vi "Main.vi"() -> ()   [LabVIEW 2020]
uses:
  <vilib>/Utility/error.llb/DialogType.ctl
  Controls/Core def.ctl
  Controls/JSON image def.ctl
  Controls/State Def.ctl
  Controls/Icons def.ctl
  <vilib>/vision/Image Controls.llb/IMAQ Image.ctl
  <vilib>/vision/NI_Vision_Development_Module.lvlib
panel:
  out "Image":T1(plugin-control)
  in  "Baud":u32=115200
  in  "Port":refnum<visa-resource-name>="COM6"
  out "STM Feedback":string
  in  "Stop filter":bool
  in  "Stop process":bool
  in  "Filter":bool
  in  "Process":bool
  in  "Stop acquisition":bool
  in  "Acquire":bool
  in  "Stop program":bool
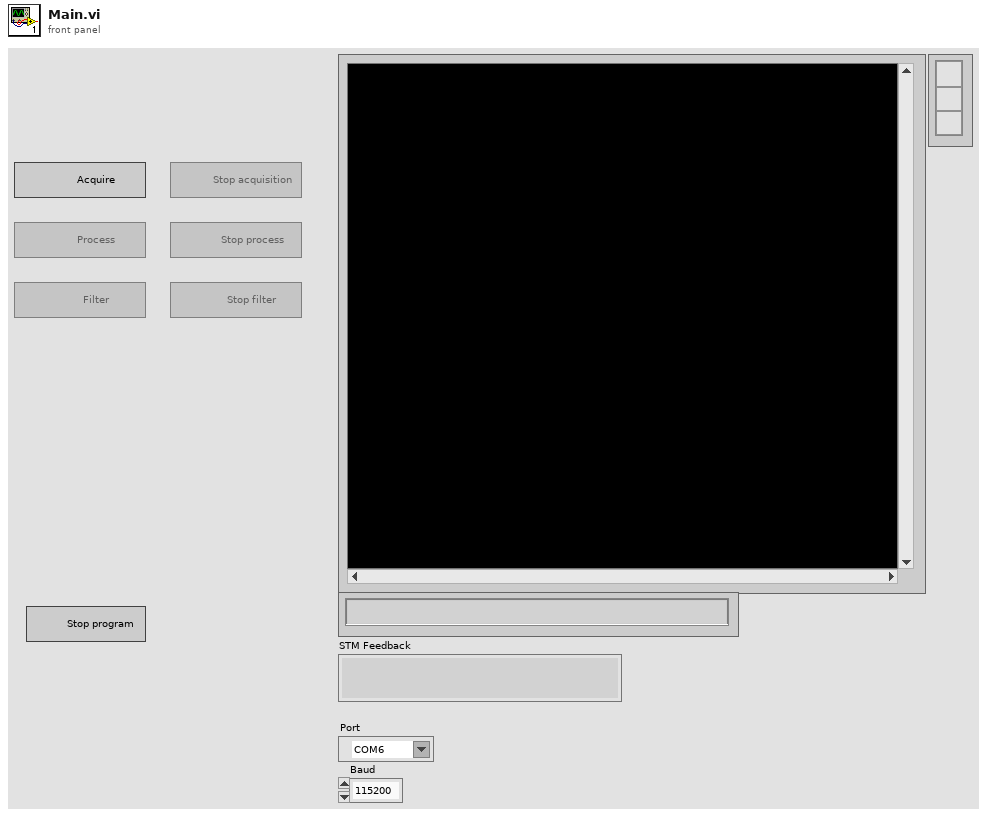
[diagram p1: front panel]
types:
  T1 = typedef "IMAQ Image.ctl" = refnum<image>
  T2 = typedef "DialogType.ctl" = u16
  T3 = enum32{"Invalid", "Standard", "Closed", "Hidden", "Minimized", "Maximized"}
  T4 = enum32{"invalid app kind", "Development System", "Run Time System", "Student Edition", "Embedded LabVIEW", "Evaluation", "Custom"}
  T5 = typedef "Icons def.ctl" = cluster{"Acquire":refnum<vi>, "Process":refnum<vi>, "Filter":refnum<vi>, "Stop acquisition":refnum<vi>, "Stop process":refnum<vi>, "Stop filter":refnum<vi>}
  T6 = typedef "State Def.ctl" = cluster{"Acquisition":bool, "Processing":bool, "Filtering":bool}
  T7 = typedef "JSON image def.ctl" = cluster{"Image Pixels (U8)":u8[][], "Image Pixels (U8) 2":u8[][], "Image Pixels (U8) 3":u8[][], "element":i32}
  T8 = typedef "Core def.ctl" = cluster{"Current VI Reference":refnum<vi>, "Close Panel on Exit?":bool}
  T9 = cluster{"Core":T8, "State":T6, "Icons":T5, "Color":i32, "New Image":T1, "JSON string":string}
  T10 = typedef "Image Type" = u32
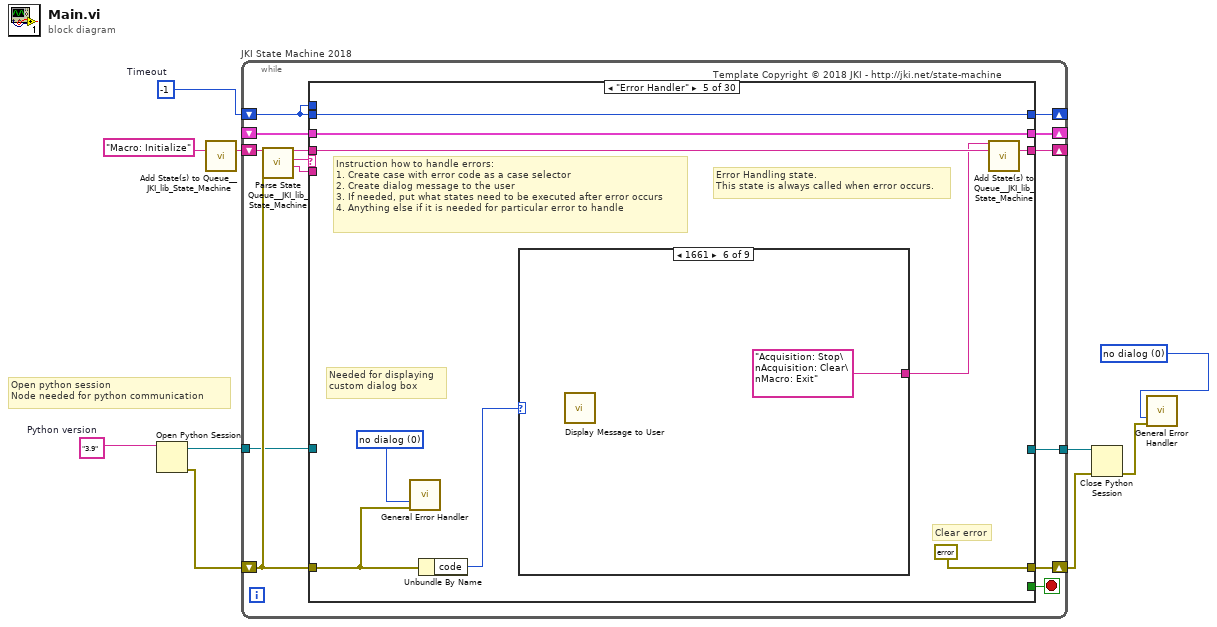
[diagram p0: block diagram]
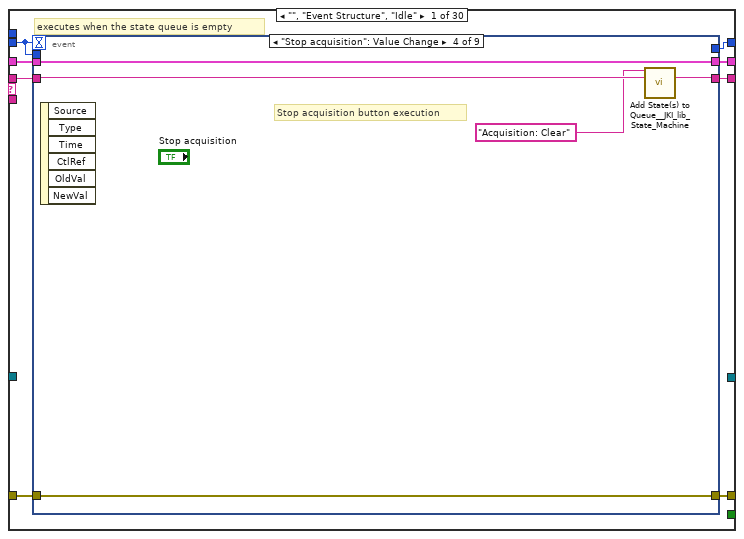
[diagram p2: hidden frame]
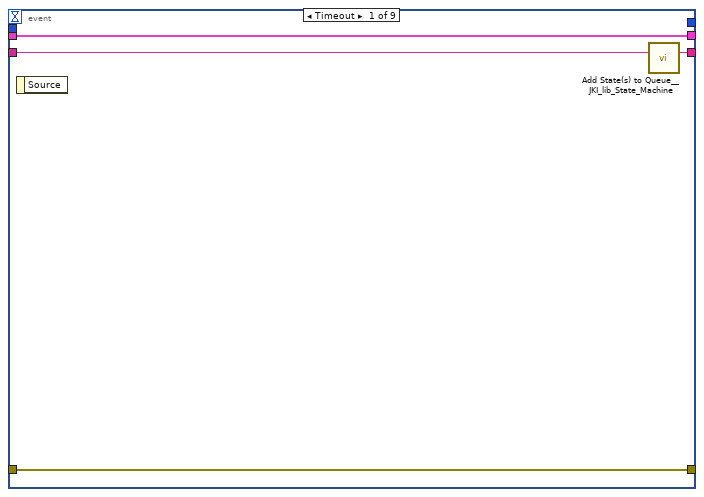
[diagram p3: hidden frame]
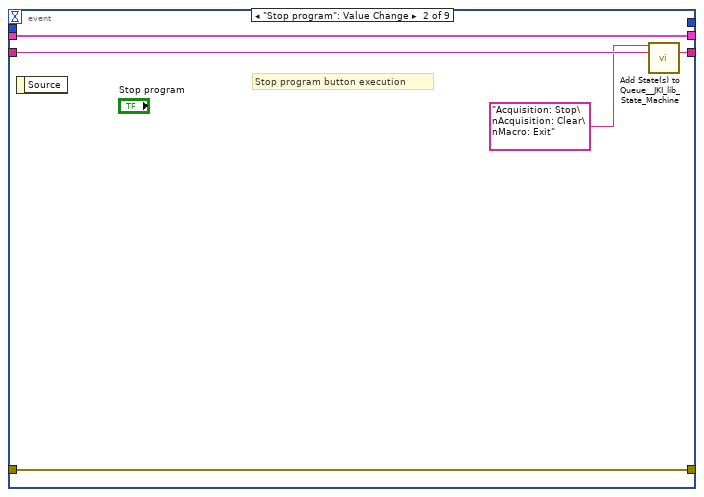
[diagram p4: hidden frame]
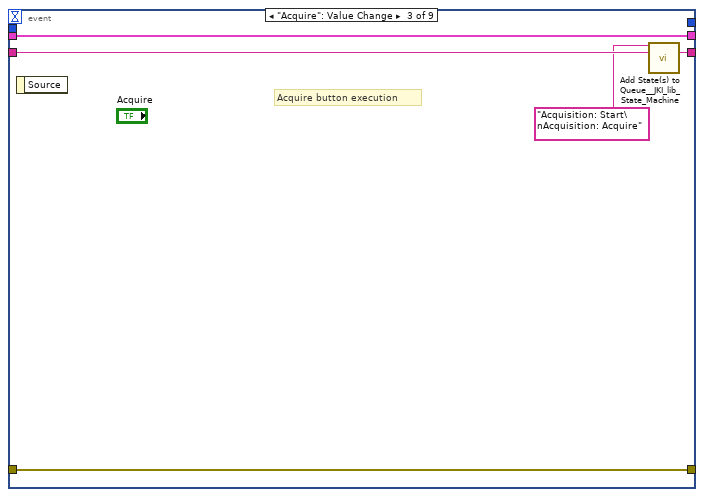
[diagram p5: hidden frame]
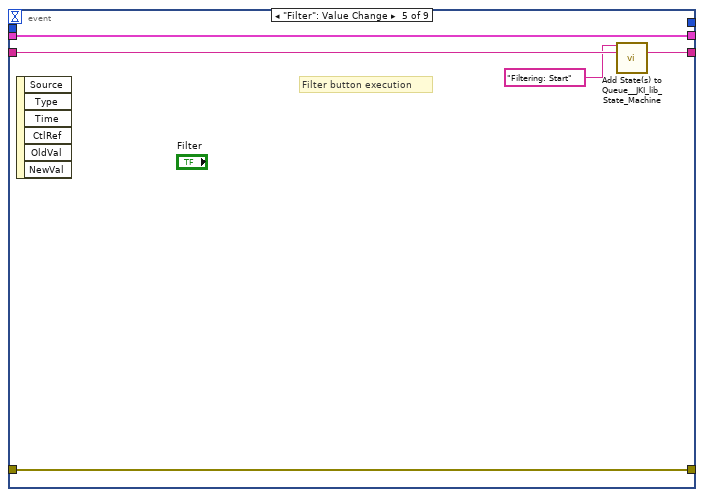
[diagram p6: hidden frame]
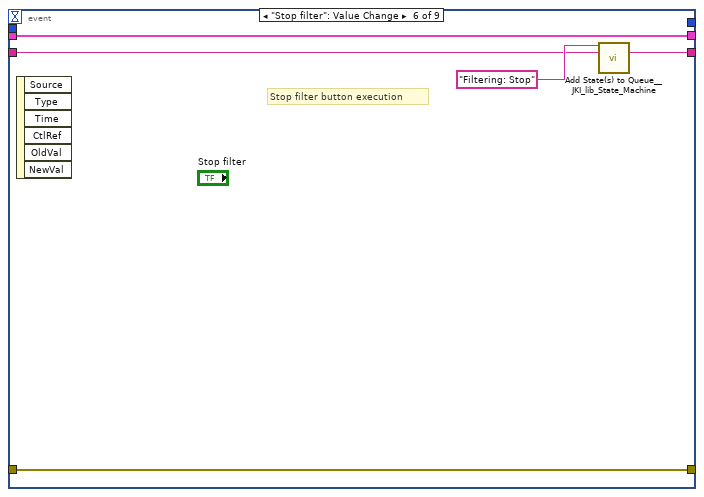
[diagram p7: hidden frame]
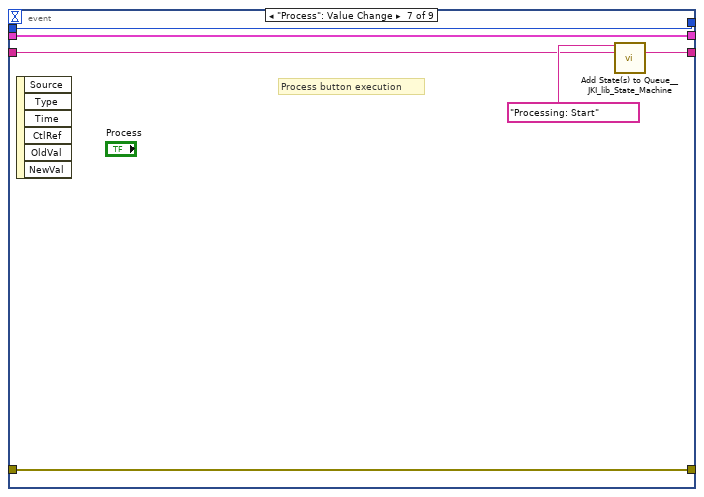
[diagram p8: hidden frame]
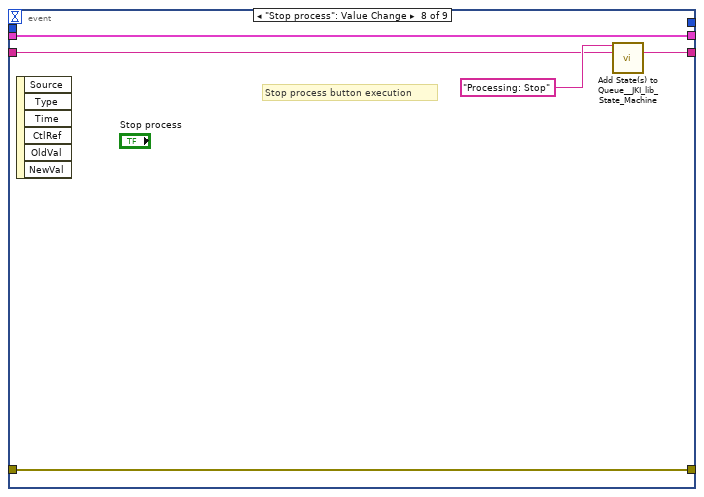
[diagram p9: hidden frame]
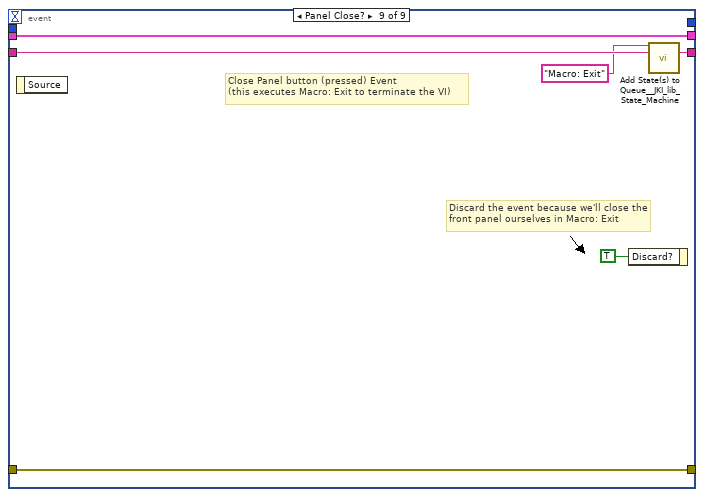
[diagram p10: hidden frame]
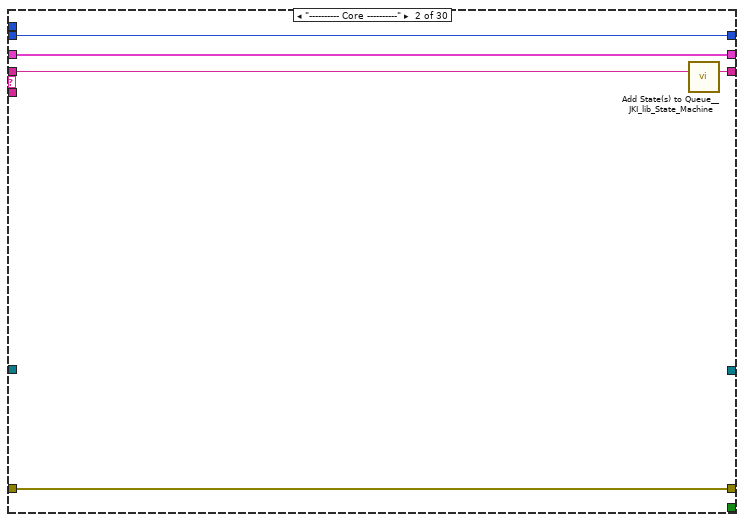
[diagram p11: hidden frame]
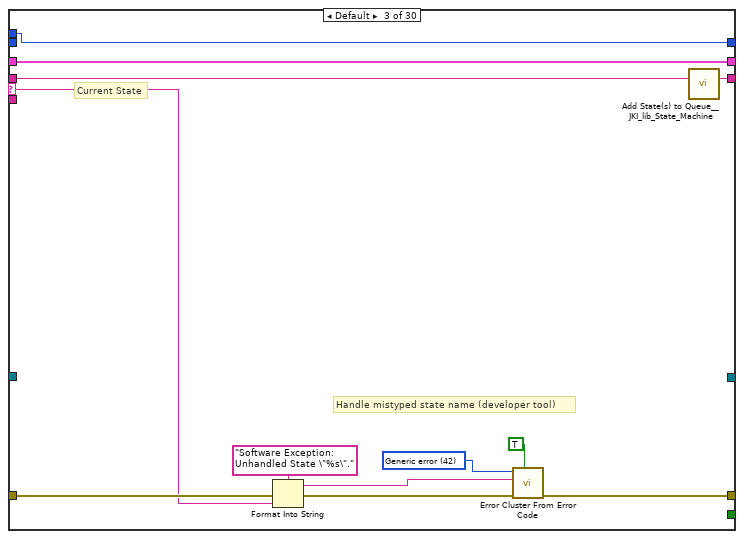
[diagram p12: hidden frame]
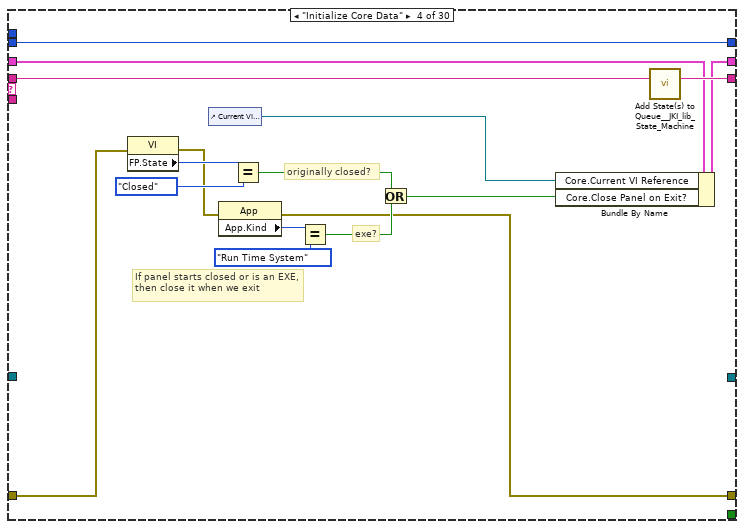
[diagram p13: hidden frame]
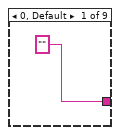
[diagram p14: hidden frame]
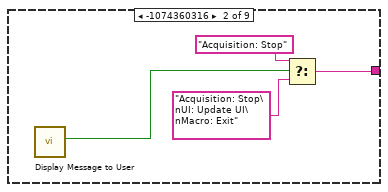
[diagram p15: hidden frame]
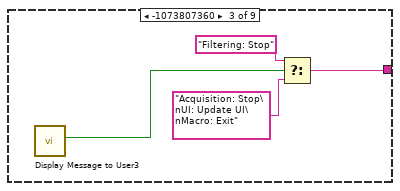
[diagram p16: hidden frame]
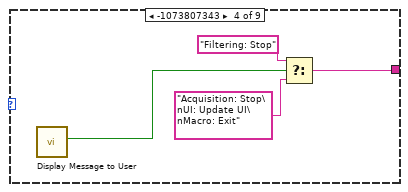
[diagram p17: hidden frame]
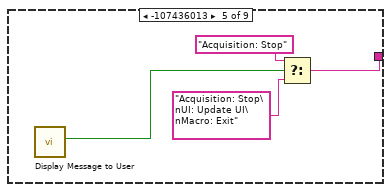
[diagram p18: hidden frame]
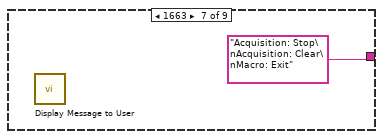
[diagram p19: hidden frame]
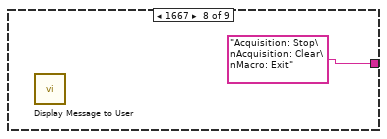
[diagram p20: hidden frame]
diagram:
  w2 = T2 0 items=["no dialog", "OK message", "continue or stop message", "OK message + warnings", "continue/stop + warnings"] ("type of dialog (OK msg:1)")
  w6 = "3.9"  # Python version
  w8 = -1  # Timeout
  # "Open python session\nNode needed for python communication"
  n1 = Open Python Session(python version=w6) -> (session out=w7:refnum<k35>, error out=w5:errorcluster)  [unwired: 2 in]
  n2 = call <vilib>:"Add State(s) to Queue__JKI_lib_State_Machine.vi"("State(s) in (\"\")"="Macro: Initialize") -> ("States Out"=w10:string)  [unwired: 14 in]
  n3 = while "JKI State Machine 2018" {
    shift-right: [w17] -> _
    shift-left: _ -> [w16]
    shift-right: [w20] -> w4
    shift-left: w5 -> [w15]
    shift-right: [w19] -> _
    shift-left: w10 -> [w21]
    shift-right: [w14] -> _
    shift-left: w8 -> [w13]
    tunnel: w7 -> [w12]
    tunnel: [w11] -> w3
    stop <- w18 stop-if-true
    # "Template Copyright © 2018 JKI - http://jki.net/state-machine"
    n4 = call <vilib>:"Parse State Queue__JKI_lib_State_Machine.vi"("State Queue"=w21, "Error In (no error)"=w15) -> ("Remaining States"=w23:string, "Current State"=w24:string, "Arguments"=w22:string)  [unwired: 11 in]
    n5 = case shown="\"Error Handler\"" w24 {
      selector: w24 -> [_ _ w85 _ _ _ _ _ _ _ _ _ _ _ _ _ _ _ _ _ _ _ _ _ _ _ _ _ _ _]
      tunnel: w23 -> [w32 w83 w89 w111 w120 w151 w156 w178 w185 w190 w205 w214 w221 w233 w298 w304 w315 w320 w334 w353 w372 w381 w386 w400 w413 w429 w434 w447 w458 w471]
      tunnel: w22 -> [_ _ _ _ _ _ _ _ _ _ _ _ w216 w227 _ _ _ _ _ _ _ _ _ _ _ _ _ _ _ _]
      tunnel: w16 -> [w30 w80 w87 w105 w117 w149 w153 _ w181 w187 w201 w207 w219 w229 w295 w301 w312 w317 w330 w351 w368 w377 w383 w397 w410 w425 w431 w443 w455 w466]
      tunnel: [w29 w81 w91 w96 errorcluster {"status"=FALSE, "code"=0, "source"=""} ("error out") w148 w154 w167 w182 w188 w203 w212 w217 w230 w296 w302 w313 w318 w332 w339 w370 w379 w384 w387 w406 w427 w432 w445 w448 w469] -> w20
      tunnel: w15 -> [w28 w81 w90 w98 w114 w148 w154 w172 w183 w188 w203 w212 w218 w231 w296 w302 w313 w318 w332 w349 w370 w379 w384 w387 w407 w427 w432 w445 w449 w469]
      tunnel: [w31 w82 w88 w110 w119 w150 w155 w177 w184 w189 w204 w213 w220 w232 w297 w303 w314 w319 w333 w352 w371 w380 w385 w399 w412 w428 w433 w446 w457 w470] -> w19
      tunnel: [_ _ _ _ _ TRUE _ _ _ _ _ _ _ _ _ _ _ _ _ _ _ _ _ _ _ _ _ _ _ _] -> w18
      tunnel: [w27 w80 w87 w109 w117 w149 w153 w157 w181 w187 w201 w207 w219 w229 w295 w301 w312 w317 w328 w343 w354 w377 w383 w395 w409 w422 w431 w435 w455 w459] -> w17
      tunnel: w13 -> [w25 w79 _ w100 w116 w146 w152 w174 w180 w186 w202 w211 w215 w226 w294 w299 w306 w316 w329 w350 w369 w378 w382 w398 w411 w426 w430 w444 w456 w468]
      tunnel: [w26 w79 w84 w100 w116 w146 w152 w174 w180 w186 w202 w211 w215 w226 w294 w299 w306 w316 w329 w350 w369 w378 w382 w398 w411 w426 w430 w444 w456 w468] -> w14
      tunnel: w13 -> [_ _ w84 _ _ _ _ _ _ _ _ _ _ _ _ _ _ _ _ _ _ _ _ _ _ _ _ _ _ _]
      tunnel: w12 -> [_ _ _ _ _ w145 _ _ _ _ _ _ _ _ _ _ _ _ _ _ _ _ _ _ w408 _ _ _ _ _]
      tunnel: [_ _ _ _ _ w145 _ _ _ _ _ _ _ _ _ _ _ _ _ _ _ _ _ _ w403 _ _ _ _ _] -> w11
      frame "", "Event Structure", "Idle" {
        # "executes when the state queue is empty"
        n6 = event shown="[3] \"Stop acquisition\": Value Change" {
          selector: _ -> [_ _ _ _ _ _ _ _ _]
          dyn-events: _ -> [_ _ _ _ _ _ _ _ _]
          timeout: w25 -> [_ _ _ _ _ _ _ _ _]
          tunnel: w32 -> [w36 w41 w46 w50 w54 w57 w62 w68 w78]
          tunnel: [w35 w40 w45 w51 w55 w59 w66 w70 w77] -> w31
          tunnel: w30 -> [w33 w38 w43 w48 w56 w61 w67 w72 w75]
          tunnel: [w34 w39 w44 w47 w52 w60 w63 w71 w76] -> w29
          tunnel: w28 -> [w34 w39 w44 w47 w52 w60 w63 w71 w76]
          tunnel: [w33 w38 w43 w48 w56 w61 w67 w72 w75] -> w27
          tunnel: [_ _ _ _ _ _ w64 _ _] -> w26
          tunnel: w25 -> [_ _ _ _ _ _ w64 _ _]
          event Timeout {
            n7 = event-data() -> ()  [unwired: 1 in, 1 out]
            n8 = call <vilib>:"Add State(s) to Queue__JKI_lib_State_Machine.vi"("State(s) in (\"\")"=w36) -> ("States Out"=w35:string)  [unwired: 14 in]
          }
          event "Stop program": Value Change {
            # "Stop program button execution"
            n9 = event-data() -> ()  [unwired: 1 in, 1 out]
            n10 = call <vilib>:"Add State(s) to Queue__JKI_lib_State_Machine.vi"("State(s) in Front (\"\")"="Acquisition: Stop\nAcquisition: Clear\nMacro: Exit", "State(s) in (\"\")"=w41) -> ("States Out"=w40:string)  [unwired: 13 in]
          }
          event "Acquire": Value Change {
            # "Acquire button execution"
            n11 = event-data() -> ()  [unwired: 1 in, 1 out]
            n12 = call <vilib>:"Add State(s) to Queue__JKI_lib_State_Machine.vi"("State(s) in Front (\"\")"="Acquisition: Start\nAcquisition: Acquire", "State(s) in (\"\")"=w46) -> ("States Out"=w45:string)  [unwired: 13 in]
          }
          event "Stop acquisition": Value Change {
            # "Stop acquisition button execution"
            n13 = event-data() -> ()  [unwired: 1 in, 6 out]
            n14 = call <vilib>:"Add State(s) to Queue__JKI_lib_State_Machine.vi"("State(s) in Front (\"\")"="Acquisition: Clear" ("State(s) in Front (\"\")"), "State(s) in (\"\")"=w50) -> ("States Out"=w51:string)  [unwired: 13 in]
          }
          event "Filter": Value Change {
            # "Filter button execution"
            n15 = event-data() -> ()  [unwired: 1 in, 6 out]
            n16 = call <vilib>:"Add State(s) to Queue__JKI_lib_State_Machine.vi"("State(s) in Front (\"\")"="Filtering: Start" ("State(s) in Front (\"\")"), "State(s) in (\"\")"=w54) -> ("States Out"=w55:string)  [unwired: 13 in]
          }
          event "Stop filter": Value Change {
            # "Stop filter button execution"
            n17 = event-data() -> ()  [unwired: 1 in, 6 out]
            n18 = call <vilib>:"Add State(s) to Queue__JKI_lib_State_Machine.vi"("State(s) in Front (\"\")"="Filtering: Stop" ("State(s) in Front (\"\")"), "State(s) in (\"\")"=w57) -> ("States Out"=w59:string)  [unwired: 13 in]
          }
          event "Process": Value Change {
            # "Process button execution"
            n19 = event-data() -> ()  [unwired: 1 in, 6 out]
            n20 = call <vilib>:"Add State(s) to Queue__JKI_lib_State_Machine.vi"("State(s) in Front (\"\")"="Processing: Start" ("State(s) in Front (\"\")"), "State(s) in (\"\")"=w62) -> ("States Out"=w66:string)  [unwired: 13 in]
          }
          event "Stop process": Value Change {
            # "Stop process button execution"
            n21 = event-data() -> ()  [unwired: 1 in, 6 out]
            n22 = call <vilib>:"Add State(s) to Queue__JKI_lib_State_Machine.vi"("State(s) in Front (\"\")"="Processing: Stop" ("State(s) in Front (\"\")"), "State(s) in (\"\")"=w68) -> ("States Out"=w70:string)  [unwired: 13 in]
          }
          event Panel Close? {
            # "Discard the event because we'll close the front panel ourselves in Macro: Exit"
            # "Close Panel button (pressed) Event\n(this executes Macro: Exit to terminate the VI)"
            n23 = event-data() -> ()  [unwired: 1 in, 1 out]
            n24 = event-data ("Event Filter Node")("Discard?"=TRUE) -> ()  [unwired: 1 in, 1 out]
            n25 = call <vilib>:"Add State(s) to Queue__JKI_lib_State_Machine.vi"("State(s) in Front (\"\")"="Macro: Exit", "State(s) in (\"\")"=w78) -> ("States Out"=w77:string)  [unwired: 13 in]
          }
        }
      }
      frame "---------- Core ----------" {
        n26 = call <vilib>:"Add State(s) to Queue__JKI_lib_State_Machine.vi"("State(s) in (\"\")"=w83) -> ("States Out"=w82:string)  [unwired: 14 in]
      }
      frame Default {
        w94 = 42 items=["No error", "Argument error", "Memory is full", "Out of zone", "End of file", "File already open", "Generic file I/O error", "File not found", "File permission error", "Disk is full", "Duplicate path", "Too many files open", "System feature not enabled", "Resource file not found", "Cannot add resource", "Resource not found", "Image not found", "Image memory error", "Pen does not exist", "Config type invalid", "Config token not found", "Config parse error", "Config memory error", "Bad external code format", "Bad external code offset", "External code not present", "Null window", "Destroy window error", "Null menu", "Print aborted", "Bad print record", "Print driver error", "Windows error during printing", "Memory error during printing", "Print dialog error", "Generic print error", "Invalid device refnum", "Device not found", "Device parameter error", "Device unit error", "Cannot open device", "Device call aborted", "Generic error", "Cancelled by user", "Object ID too low", "Object ID too high", "Object not in heap", "Unknown heap", "Unknown object (invalid DefProc)", "Unknown object (DefProc not in table)", "Message out of range", "Invalid (null) method", "Unknown message", "Manager call not supported", "Bad address", "Network operation in progress", "Network operation timed out", "Connection is busy", "Network attribute not supported", "Network error", "Address in use", "System out of memory", "Connection aborted", "Connection refused", "Not connected", "Already connected", "Connection closed", "Initialization error (interapplication manager)", "Bad occurrence", "Wait on unbound occurrence handler", "Occurrence queue overflow", "Datalog type conflict", "Unused", "Unrecognized type (interapplication manager)", "Memory corrupt", "Failed to make temporary DLL", "Old CIN version", "Drag socket not found", "Failed to load drop-object", "Failed to register OLE object", "Failed to release OLE object", "Format specifier type mismatch", "Unknown format specifier", "Too few format specifiers", "Too many format specifiers", "Scan failed", "Newer CIN version", "Error converting to variant", "Runtime menu error", "Password tampered", "Variant attribute not found", "Incompatible variant data type", "Event data is not available", "Event Store is not present", "Occurrence is not found", "Event Queue is not created", "Event info is not available", "Refnum passed is NULL", "Error retrieving Class GUID", "Error retrieving CoClass GUID", "Error retrieving TypeLib GUID.", "Bad built application magic bytes.", "Specific driver is different from the specific driver associated with the Logical Name.", "There is no session opened to the class driver.", "Max Error", "MAX - Error with config objects", "MAX - Error loading configuration", "MAX - Group not supported"]
        # "Current State"
        # "Handle mistyped state name (developer tool)"
        n27 = Format Into String(format string="Software Exception: Unhandled State \"%s\"." ("message"), error in=w90, w85) -> (resulting string=w93:string, error out=w92:errorcluster)  [unwired: 1 in]
        n28 = call <vilib>:"Error Cluster From Error Code.vi"("show call chain? (False)"=TRUE, "error in (no error)"=w92, "error message (\"\")"=w93, "error code (0)"=w94) -> ("error out"=w91:errorcluster)  [unwired: 5 in]
        n29 = call <vilib>:"Add State(s) to Queue__JKI_lib_State_Machine.vi"("State(s) in (\"\")"=w89) -> ("States Out"=w88:string)  [unwired: 14 in]
      }
      frame "Initialize Core Data" {
        # "originally closed?"
        # "exe?"
        # "If panel starts closed or is an EXE, then close it when we exit"
        n30 = property on="Property Node" class="VI"(error in=w98) -> (error out=w97:errorcluster, "FP.State"=w103:T3)  [unwired: 1 in, 1 out]
        n31 = control-ref of="Current VI Reference"() -> (w104:refnum<vi>)
        n32 = property on="Property Node" class="App"(error in=w97) -> (error out=w96:errorcluster, "App.Kind"=w108:T4)  [unwired: 1 in, 1 out]
        n33 = Equal?(x=w103, y=T3."Closed" ("Front Panel Window:State")) -> (x = y?=w101:bool)
        n34 = Equal?(x=w108, y=T4."Run Time System" ("Application:Kind")) -> (x = y?=w106:bool)
        n35 = Or(x=w101, y=w106) -> (x .or. y?=w99:bool)
        n36 = Bundle By Name(cluster=w105, "Core.Current VI Reference"=w104, "Core.Close Panel on Exit?"=w99) -> (w109:T9)
        n37 = call <vilib>:"Add State(s) to Queue__JKI_lib_State_Machine.vi"("State(s) in (\"\")"=w111) -> ("States Out"=w110:string)  [unwired: 14 in]
      }
      frame "Error Handler" {
        w113 = T2 0 items=["no dialog", "OK message", "continue or stop message", "OK message + warnings", "continue/stop + warnings"] ("type of dialog (OK msg:1)")
        # "Needed for displaying\ncustom dialog box"
        # "Instruction how to handle errors:\n1. Create case with error code as a case selector\n2. Create dialog message to the user\n3. If needed, put what states need to be executed after error occurs\n4. Anything else if it is needed for particular error to handle"
        # "Error Handling state.\nThis state is always called when error occurs."
        # "Clear error"
        n38 = call <vilib>:"General Error Handler.vi"("type of dialog (OK msg:1)"=w113, "error in (no error)"=w114) -> ()  [unwired: 9 in, 5 out]
        n39 = Unbundle By Name(w114) -> ("code"=w115:i32)
        n40 = case shown="1661" w115 {
          tunnel: ["" w122 w126 w130 w134 "Acquisition: Stop\nAcquisition: Clear\nMacro: Exit" "Acquisition: Stop\nAcquisition: Clear\nMacro: Exit" "Acquisition: Stop\nAcquisition: Clear\nMacro: Exit" w142] -> w112
          frame 0, Default {
          }
          frame -1074360316 {
            n41 = call "Display Message to User"() -> ("Continue"=w125:bool)  [unwired: 10 in, 1 out]
            n42 = Select(t="Acquisition: Stop", s=w125, f="Acquisition: Stop\nUI: Update UI\nMacro: Exit") -> (s? t:f=w122:string)
          }
          frame -1073807360 {
            n43 = call "Display Message to User3"() -> ("Continue"=w129:bool)  [unwired: 10 in, 1 out]
            n44 = Select(t="Filtering: Stop", s=w129, f="Acquisition: Stop\nUI: Update UI\nMacro: Exit") -> (s? t:f=w126:string)
          }
          frame -1073807343 {
            n45 = call "Display Message to User"() -> ("Continue"=w133:bool)  [unwired: 10 in, 1 out]
            n46 = Select(t="Filtering: Stop", s=w133, f="Acquisition: Stop\nUI: Update UI\nMacro: Exit") -> (s? t:f=w130:string)
          }
          frame -107436013 {
            n47 = call "Display Message to User"() -> ("Continue"=w137:bool)  [unwired: 10 in, 1 out]
            n48 = Select(t="Acquisition: Stop", s=w137, f="Acquisition: Stop\nUI: Update UI\nMacro: Exit") -> (s? t:f=w134:string)
          }
          frame 1661 {
            n49 = call "Display Message to User"() -> ()  [unwired: 10 in, 2 out]
          }
          frame 1663 {
            n50 = call "Display Message to User"() -> ()  [unwired: 10 in, 2 out]
          }
          frame 1667 {
            n51 = call "Display Message to User"() -> ()  [unwired: 10 in, 2 out]
          }
          frame 1073676294 {
            # "If you want to see this error handling in action, just hard-code code of error as 1073676294 in any state."
            # "Tip: Decision making is not necessary. If particular error needs to be handled in only one way, just output states needed to be executed to handle error properly and disable second button in Display Message to User."
            # "Decision making depending\non what button user clicks."
            # "Custom dialog box"
            n52 = call "Display Message to User"() -> ("Continue"=w144:bool)  [unwired: 10 in, 1 out]
            n53 = Select(t="Filtering: Stop", s=w144, f="Acquisition: Stop\nUI: Update UI\nMacro: Exit") -> (s? t:f=w142:string)
          }
        }
        n54 = call <vilib>:"Add State(s) to Queue__JKI_lib_State_Machine.vi"("State(s) in Front (\"\")"=w112, "State(s) in (\"\")"=w120) -> ("States Out"=w119:string)  [unwired: 13 in]
      }
      frame "Exit" {
        n55 = call <vilib>:"Add State(s) to Queue__JKI_lib_State_Machine.vi"("State(s) in (\"\")"=w151) -> ("States Out"=w150:string)  [unwired: 14 in]
      }
      frame "---------- Data ----------" {
        n56 = call <vilib>:"Add State(s) to Queue__JKI_lib_State_Machine.vi"("State(s) in (\"\")"=w156) -> ("States Out"=w155:string)  [unwired: 14 in]
      }
      frame "Data: Initialize" {
        w173 = 0  # Color
        # "Here all data is initialized and bundle'd into cluster"
        n57 = control-ref of="Acquire"() -> (w164:refnum<vi>)
        n58 = control-ref of="Process"() -> (w163:refnum<vi>)
        n59 = control-ref of="Filter"() -> (w162:refnum<vi>)
        n60 = control-ref of="Stop acquisition"() -> (w161:refnum<vi>)
        n61 = control-ref of="Stop process"() -> (w160:refnum<vi>)
        n62 = control-ref of="Stop filter"() -> (w159:refnum<vi>)
        n63 = Bundle By Name(cluster=T5 {"Acquire"=refnum, "Process"=refnum, "Filter"=refnum, "Stop acquisition"=refnum, "Stop process"=refnum, "Stop filter"=refnum} ("Icons"), "Acquire"=w164, "Process"=w163, "Filter"=w162, "Stop acquisition"=w161, "Stop process"=w160, "Stop filter"=w159) -> (w158:T5)
        n64 = call "IMAQ Create"("Image Name"="processed_image", "error in (no error)"=w172) -> ("New Image"=w169:T1, "error out"=w171:errorcluster)  [unwired: 3 in]
        n65 = Flatten To JSON(anything=T7 {"Image Pixels (U8)"=[], "Image Pixels (U8) 2"=[], "Image Pixels (U8) 3"=[], "element"=0}, error in (no error)=w171) -> (JSON string=w168:string, 11:w167:errorcluster)  [unwired: 1 in]
        n66 = Bundle("Core"=T8 {"Current VI Reference"=refnum, "Close Panel on Exit?"=FALSE}, "State"=T6 {"Acquisition"=FALSE, "Processing"=FALSE, "Filtering"=FALSE}, "Icons"=w158, "Color"=w173, "New Image"=w169, "JSON string"=w168) -> (w157:T9)  [unwired: 1 in]
        n67 = call <vilib>:"Add State(s) to Queue__JKI_lib_State_Machine.vi"("State(s) in (\"\")"=w178) -> ("States Out"=w177:string)  [unwired: 14 in]
      }
      frame "Data: Cleanup" {
        n68 = Unbundle By Name(w181) -> ("Core.Current VI Reference"=w179:refnum<vi>)
        n69 = Close Reference(reference=w179, error in (no error)=w183) -> (error out=w182:errorcluster)
        n70 = call <vilib>:"Add State(s) to Queue__JKI_lib_State_Machine.vi"("State(s) in (\"\")"=w185) -> ("States Out"=w184:string)  [unwired: 14 in]
      }
      frame "---------- UI ----------" {
        n71 = call <vilib>:"Add State(s) to Queue__JKI_lib_State_Machine.vi"("State(s) in (\"\")"=w190) -> ("States Out"=w189:string)  [unwired: 14 in]
      }
      frame "UI: Initialize" {
        # "This state is called only at the program setup stage.\nIt sets front panel icons to default state."
        n72 = Unbundle By Name(w201) -> ("Icons.Acquire"=w193:refnum<vi>, "Icons.Process"=w200:refnum<vi>, "Icons.Filter"=w199:refnum<vi>, "Icons.Stop acquisition"=w196:refnum<vi>, "Icons.Stop process"=w198:refnum<vi>, "Icons.Stop filter"=w197:refnum<vi>)
        n73 = Build Array(w193) -> (w192:refnum<vi>[])
        n74 = Build Array(w200, w199, w196, w198, w197) -> (w194:refnum<vi>[])
        n75 = call "Set Enable State on Multiple Controls.vi"("Enable?"=TRUE, "Controls"=w192) -> ()  [unwired: 10 in]
        n76 = call "Set Enable State on Multiple Controls.vi"("Enable?"=FALSE, "Controls"=w194) -> ()  [unwired: 10 in]
        n77 = call <vilib>:"Add State(s) to Queue__JKI_lib_State_Machine.vi"("State(s) in (\"\")"=w205) -> ("States Out"=w204:string)  [unwired: 14 in]
      }
      frame "UI: Update UI" {
        # "If acquisition is OFF, clear image"
        # "If acquisition is ON, update image"
        # "Here image is updated"
        n78 = Unbundle By Name(w207) -> ("State.Acquisition"=w208:bool)
        n79 = Unbundle By Name(w207) -> ("New Image"=w210:T1)
        n80 = Select(t=w210, s=w208, f=T1 refnum ("t")) -> (s? t:f=→"Image":T1)
        n81 = call <vilib>:"Add State(s) to Queue__JKI_lib_State_Machine.vi"("State(s) in (\"\")"=w214) -> ("States Out"=w213:string)  [unwired: 14 in]
      }
      frame "UI: Cursor Set" {
        # "Argument"
        n82 = case shown="\"Idle\", Default" w216 {
          tunnel: w218 -> [w223 w225]
          tunnel: [w222 w224] -> w217
          frame "Idle", Default {
            n83 = call <vilib>:"Unset Busy.vi"("error in (no error)"=w223) -> ("error out"=w222:errorcluster)  [unwired: 10 in]
          }
          frame "Busy" {
            n84 = call <vilib>:"Set Busy.vi"("error in (no error)"=w225) -> ("error out"=w224:errorcluster)  [unwired: 9 in, 1 out]
          }
        }
        n85 = call <vilib>:"Add State(s) to Queue__JKI_lib_State_Machine.vi"("State(s) in (\"\")"=w221) -> ("States Out"=w220:string)  [unwired: 14 in]
      }
      frame "UI: Front Panel State" {
        # "Argument"
        n86 = Unbundle By Name(w229) -> ("Core.Current VI Reference"=w228:refnum<vi>)
        n87 = case shown="\"Close\", \"Closed\"" w227 {
          tunnel: w231 -> [w239 w252 w263 w275 w287]
          tunnel: [w240 w253 w264 w276 w288] -> w230
          tunnel: w228 -> [_ _ _ _ _]
          frame "Open", "Standard", Default {
            w234 = T3."Standard" ("State")
            n88 = property on="Property Node" class="VI"(error in=w239) -> (reference out=w237:refnum<vi>, error out=w238:errorcluster, "FP.State"=w236:T3)  [unwired: 1 in]
            n89 = Not Equal?(x=w236, y=w234) -> (x != y?=w235:bool)
            n90 = case shown="True" w235 {
              tunnel: [w244 w246] -> w240
              tunnel: w238 -> [w243 w246]
              tunnel: w237 -> [w242 _]
              tunnel: w234 -> [w241 _]
              frame True {
                n91 = invoke on="Invoke Node" class="VI" method="FP.Open"(reference=w242, error in=w243, "Activate"=TRUE, "State"=w241) -> (error out=w244:errorcluster)  [unwired: 1 in, 4 out]
              }
              frame False {
              }
            }
          }
          frame "Close", "Closed" {
            n92 = property on="Property Node" class="VI"(error in=w252) -> (reference out=w250:refnum<vi>, error out=w251:errorcluster, "FP.State"=w248:T3)  [unwired: 1 in]
            n93 = Not Equal?(x=w248, y=T3."Closed" ("Front Panel Window:State")) -> (x != y?=w247:bool)
            n94 = case shown="True" w247 {
              tunnel: [w254 w257] -> w253
              tunnel: w251 -> [w254 w256]
              tunnel: w250 -> [_ w255]
              frame False {
              }
              frame True {
                n95 = invoke on="Invoke Node" class="VI" method="FP.Close"(reference=w255, error in=w256) -> (error out=w257:errorcluster)  [unwired: 1 in, 2 out]
              }
            }
          }
          frame "Hidden", "Hide" {
            w258 = T3."Hidden" ("State")
            n96 = property on="Property Node" class="VI"(error in=w263) -> (reference out=w261:refnum<vi>, error out=w262:errorcluster, "FP.State"=w260:T3)  [unwired: 1 in]
            n97 = Not Equal?(x=w260, y=w258) -> (x != y?=w259:bool)
            n98 = case shown="True" w259 {
              tunnel: [w268 w269] -> w264
              tunnel: w262 -> [w267 w269]
              tunnel: w261 -> [w266 _]
              tunnel: w258 -> [w265 _]
              frame True {
                n99 = invoke on="Invoke Node" class="VI" method="FP.Open"(reference=w266, error in=w267, "State"=w265) -> (error out=w268:errorcluster)  [unwired: 2 in, 4 out]
              }
              frame False {
              }
            }
          }
          frame "Minimize", "Minimized" {
            w270 = T3."Minimized" ("State")
            n100 = property on="Property Node" class="VI"(error in=w275) -> (reference out=w273:refnum<vi>, error out=w274:errorcluster, "FP.State"=w272:T3)  [unwired: 1 in]
            n101 = Not Equal?(x=w272, y=w270) -> (x != y?=w271:bool)
            n102 = case shown="True" w271 {
              tunnel: [w280 w281] -> w276
              tunnel: w274 -> [w279 w281]
              tunnel: w273 -> [w278 _]
              tunnel: w270 -> [w277 _]
              frame True {
                n103 = invoke on="Invoke Node" class="VI" method="FP.Open"(reference=w278, error in=w279, "State"=w277) -> (error out=w280:errorcluster)  [unwired: 2 in, 4 out]
              }
              frame False {
              }
            }
          }
          frame "Maximize", "Maximized" {
            w282 = T3."Maximized" ("State")
            n104 = property on="Property Node" class="VI"(error in=w287) -> (reference out=w285:refnum<vi>, error out=w286:errorcluster, "FP.State"=w284:T3)  [unwired: 1 in]
            n105 = Not Equal?(x=w284, y=w282) -> (x != y?=w283:bool)
            n106 = case shown="True" w283 {
              tunnel: [w292 w293] -> w288
              tunnel: w286 -> [w291 w293]
              tunnel: w285 -> [w290 _]
              tunnel: w282 -> [w289 _]
              frame True {
                n107 = invoke on="Invoke Node" class="VI" method="FP.Open"(reference=w290, error in=w291, "State"=w289) -> (error out=w292:errorcluster)  [unwired: 2 in, 4 out]
              }
              frame False {
              }
            }
          }
        }
        n108 = call <vilib>:"Add State(s) to Queue__JKI_lib_State_Machine.vi"("State(s) in (\"\")"=w233) -> ("States Out"=w232:string)  [unwired: 14 in]
      }
      frame "---------- Macro ----------" {
        n109 = call <vilib>:"Add State(s) to Queue__JKI_lib_State_Machine.vi"("State(s) in (\"\")"=w298) -> ("States Out"=w297:string)  [unwired: 14 in]
      }
      frame "Macro: Initialize" {
        w300 = "Data: Initialize\nInitialize Core Data\nUI: Initialize\nUI: Front Panel State >> Open"  # Data: Initialize Initialize Core Data UI: Initialize UI: Front Panel State >> Open
        # "This state runs at setup stage\nIt holds states to run at setup stage"
        n110 = call <vilib>:"Add State(s) to Queue__JKI_lib_State_Machine.vi"("State(s) in Front (\"\")"=w300, "State(s) in (\"\")"=w304) -> ("States Out"=w303:string)  [unwired: 13 in]
      }
      frame "Macro: Exit" {
        # "This state runs when program gets order to exit"
        n111 = Unbundle By Name(w312) -> ("Core.Close Panel on Exit?"=w305:bool)
        n112 = Select(t="UI: Front Panel State >> Close", s=w305, f="" ("Empty String Constant")) -> (s? t:f=w309:string)
        n113 = call <vilib>:"Add State(s) to Queue__JKI_lib_State_Machine.vi"("State(s) in (\"\")"=w309, "State(s) at Back (\"\")"="Data: Cleanup\nExit") -> ("States Out"=w307:string)  [unwired: 13 in]
        n114 = call <vilib>:"Add State(s) to Queue__JKI_lib_State_Machine.vi"("State(s) in Front (\"\")"=w307, "State(s) in (\"\")"=w315) -> ("States Out"=w314:string)  [unwired: 13 in]
      }
      frame "---------- Acquisition ----------" {
        n115 = call <vilib>:"Add State(s) to Queue__JKI_lib_State_Machine.vi"("State(s) in (\"\")"=w320) -> ("States Out"=w319:string)  [unwired: 14 in]
      }
      frame "Acquisition: Start" {
        # "Enable icons"
        # "Disable icons"
        # "Changing acquisition to TRUE"
        n116 = Bundle By Name(cluster=w330, "State.Acquisition"=TRUE ("Aborted")) -> (w328:T9)
        n117 = Unbundle By Name(w328) -> ("Icons.Acquire"=w327:refnum<vi>, "Icons.Process"=w324:refnum<vi>, "Icons.Stop acquisition"=w321:refnum<vi>)
        n118 = Build Array(w327) -> (w326:refnum<vi>[])
        n119 = Build Array(w324, w321) -> (w323:refnum<vi>[])
        n120 = call "Set Enable State on Multiple Controls.vi"("Enable?"=FALSE, "Controls"=w326) -> ()  [unwired: 10 in]
        n121 = call "Set Enable State on Multiple Controls.vi"("Enable?"=TRUE, "Controls"=w323) -> ()  [unwired: 10 in]
        n122 = call <vilib>:"Add State(s) to Queue__JKI_lib_State_Machine.vi"("State(s) in (\"\")"=w334) -> ("States Out"=w333:string)  [unwired: 14 in]
      }
      frame "Acquisition: Acquire" {
        w345 = 300  # X Resolution
        w346 = 300  # Y Resolution
        w347 = T10 4 items=["Grayscale (U8)", "Grayscale (I16)", "Grayscale (SGL)", "Complex (CSG)", "RGB (U32)", "HSL (U32)", "RGB (U64)", "Grayscale (U16)"]  # Image Type
        # "Choosing states to run depending on\nAcquire, Process and Filter buttons states"
        # "Converting image representation\n and resolution"
        # "Acquire image from camera"
        n123 = call "Vision Acquisition"("error in"=w349) -> ("Image Out"=w348:T1, "error out"=w342:errorcluster)  [unwired: 24 in, 1 out]
        n124 = call "IMAQ Cast Image 2"("Image Src"=w348, "Image Type"=w347, "error in (no error)"=w342) -> ("Image Dst Out"=w341:T1, "error out"=w340:errorcluster)  [unwired: 11 in]
        n125 = call "IMAQ Resample"("X Resolution"=w345, "Y Resolution"=w346, "error in (no error)"=w340, "Image Src"=w341) -> ("error out"=w339:errorcluster, "Image Dst Out"=w338:T1)  [unwired: 6 in]
        n126 = Bundle By Name(cluster=w351, "New Image"=w338) -> (w343:T9)
        n127 = Unbundle By Name(w343) -> ("State.Acquisition"=w337:bool, "State.Processing"=w336:bool, "State.Filtering"=w335:bool)
        n128 = call "State Logic.vi"("Filtering"=w335, "Processing"=w336, "Acquisition"=w337) -> ("WhatToDo"=w344:string)  [unwired: 8 in]
        n129 = call <vilib>:"Add State(s) to Queue__JKI_lib_State_Machine.vi"("State(s) in Front (\"\")"=w344, "State(s) in (\"\")"=w353) -> ("States Out"=w352:string)  [unwired: 13 in]
      }
      frame "Acquisition: Stop" {
        # "Enable icons"
        # "Disable icons"
        # "Changing acquisition, processing and filtering to FALSE"
        n130 = Bundle By Name(cluster=w368, "State.Acquisition"=FALSE ("Aborted"), "State.Processing"=FALSE ("Processing"), "State.Filtering"=FALSE ("Filtering")) -> (w354:T9)
        n131 = Unbundle By Name(w354) -> ("Icons.Acquire"=w357:refnum<vi>, "Icons.Process"=w364:refnum<vi>, "Icons.Filter"=w363:refnum<vi>, "Icons.Stop acquisition"=w360:refnum<vi>, "Icons.Stop process"=w362:refnum<vi>, "Icons.Stop filter"=w361:refnum<vi>)
        n132 = Build Array(w357) -> (w356:refnum<vi>[])
        n133 = Build Array(w364, w363, w360, w362, w361) -> (w358:refnum<vi>[])
        n134 = call "Set Enable State on Multiple Controls.vi"("Enable?"=TRUE, "Controls"=w356) -> ()  [unwired: 10 in]
        n135 = call "Set Enable State on Multiple Controls.vi"("Enable?"=FALSE, "Controls"=w358) -> ()  [unwired: 10 in]
        n136 = call <vilib>:"Add State(s) to Queue__JKI_lib_State_Machine.vi"("State(s) in (\"\")"=w372) -> ("States Out"=w371:string)  [unwired: 14 in]
      }
      frame "Acquisition: Clear" {
        # "This state makes sure image in front panel is cleared"
        n137 = Unbundle By Name(w377) -> ("State.Acquisition"=w373:bool)
        n138 = Select(t="Acquisition: Stop", s=w373, f="UI: Update UI") -> (s? t:f=w375:string)
        n139 = call <vilib>:"Add State(s) to Queue__JKI_lib_State_Machine.vi"("State(s) in Front (\"\")"=w375, "State(s) in (\"\")"=w381) -> ("States Out"=w380:string)  [unwired: 13 in]
      }
      frame "---------- Processing ----------" {
        n140 = call <vilib>:"Add State(s) to Queue__JKI_lib_State_Machine.vi"("State(s) in (\"\")"=w386) -> ("States Out"=w385:string)  [unwired: 14 in]
      }
      frame "Processing: Start" {
        # "Disable icons"
        # "Enable icons"
        # "Changing processing to TRUE"
        n141 = Bundle By Name(cluster=w397, "State.Processing"=TRUE ("IsFaceDetectionON")) -> (w395:T9)
        n142 = Unbundle By Name(w395) -> ("Icons.Process"=w394:refnum<vi>, "Icons.Stop process"=w391:refnum<vi>, "Icons.Filter"=w390:refnum<vi>)
        n143 = Build Array(w394) -> (w393:refnum<vi>[])
        n144 = Build Array(w391, w390) -> (w389:refnum<vi>[])
        n145 = call "Set Enable State on Multiple Controls.vi"("Enable?"=FALSE, "Controls"=w393) -> ()  [unwired: 10 in]
        n146 = call "Set Enable State on Multiple Controls.vi"("Enable?"=TRUE, "Controls"=w389) -> ()  [unwired: 10 in]
        n147 = call <vilib>:"Add State(s) to Queue__JKI_lib_State_Machine.vi"("State(s) in (\"\")"=w400) -> ("States Out"=w399:string)  [unwired: 14 in]
      }
      frame "Processing: Process" {
        # "subVI that converts image, sends to python script that processes image,\nconverts back image and return processed image and found color"
        # "This state is to process image"
        n148 = Unbundle By Name(w410) -> ("New Image"=w402:T1, "JSON string"=w401:string)
        n149 = call "Process Image.vi"("error in (no error)"=w407, "session out"=w408, "JSON string"=w401, "Image in"=w402) -> ("error out"=w406:errorcluster, "session in"=w403:refnum<k35>, "Color"=w404:i32, "Image out"=w405:T1)  [unwired: 4 in]
        n150 = Bundle By Name(cluster=w410, "New Image"=w405, "Color"=w404) -> (w409:T9)
        n151 = call <vilib>:"Add State(s) to Queue__JKI_lib_State_Machine.vi"("State(s) in (\"\")"=w413) -> ("States Out"=w412:string)  [unwired: 14 in]
      }
      frame "Processing: Stop" {
        # "Disable icons"
        # "Enable icons"
        # "Changing processing and filtering to FALSE"
        n152 = Bundle By Name(cluster=w425, "State.Processing"=FALSE ("Processing"), "State.Filtering"=FALSE ("Processing")) -> (w422:T9)
        n153 = Unbundle By Name(w422) -> ("Icons.Process"=w417:refnum<vi>, "Icons.Filter"=w416:refnum<vi>, "Icons.Stop process"=w415:refnum<vi>, "Icons.Stop filter"=w414:refnum<vi>)
        n154 = Build Array(w417) -> (w421:refnum<vi>[])
        n155 = Build Array(w416, w415, w414) -> (w419:refnum<vi>[])
        n156 = call "Set Enable State on Multiple Controls.vi"("Enable?"=TRUE, "Controls"=w421) -> ()  [unwired: 10 in]
        n157 = call "Set Enable State on Multiple Controls.vi"("Enable?"=FALSE, "Controls"=w419) -> ()  [unwired: 10 in]
        n158 = call <vilib>:"Add State(s) to Queue__JKI_lib_State_Machine.vi"("State(s) in (\"\")"=w429) -> ("States Out"=w428:string)  [unwired: 14 in]
      }
      frame "---------- Filtering ----------" {
        n159 = call <vilib>:"Add State(s) to Queue__JKI_lib_State_Machine.vi"("State(s) in (\"\")"=w434) -> ("States Out"=w433:string)  [unwired: 14 in]
      }
      frame "Filtering: Start" {
        # "Changing processing to TRUE"
        # "Enable icons"
        # "Disable icons"
        n160 = Bundle By Name(cluster=w443, "State.Filtering"=TRUE ("Filtering")) -> (w435:T9)
        n161 = Unbundle By Name(w435) -> ("Icons.Filter"=w441:refnum<vi>, "Icons.Stop filter"=w438:refnum<vi>)
        n162 = Build Array(w441) -> (w440:refnum<vi>[])
        n163 = Build Array(w438) -> (w437:refnum<vi>[])
        n164 = call "Set Enable State on Multiple Controls.vi"("Enable?"=FALSE, "Controls"=w440) -> ()  [unwired: 10 in]
        n165 = call "Set Enable State on Multiple Controls.vi"("Enable?"=TRUE, "Controls"=w437) -> ()  [unwired: 10 in]
        n166 = call <vilib>:"Add State(s) to Queue__JKI_lib_State_Machine.vi"("State(s) in (\"\")"=w447) -> ("States Out"=w446:string)  [unwired: 14 in]
      }
      frame "Filtering: Filter" {
        n167 = Unbundle By Name(w455) -> ("Color"=w450:i32, "State.Filtering"=w451:bool)
        n168 = call "Sorting belt control.vi"("error in (no error)"=w449, "State.Filtering"=w451, "Color"=w450, "Baud"="Baud", "VISA Refnum in"="Port") -> ("STM Feedback"=→"STM Feedback":string, "error out"=w448:errorcluster)  [unwired: 5 in]
        n169 = call <vilib>:"Add State(s) to Queue__JKI_lib_State_Machine.vi"("State(s) in (\"\")"=w458) -> ("States Out"=w457:string)  [unwired: 14 in]
      }
      frame "Filtering: Stop" {
        # "Enable icons"
        # "Disable icons"
        # "Changing processing to FALSE"
        n170 = Bundle By Name(cluster=w466, "State.Filtering"=FALSE ("Filtering")) -> (w459:T9)
        n171 = Unbundle By Name(w459) -> ("Icons.Filter"=w465:refnum<vi>, "Icons.Stop filter"=w462:refnum<vi>)
        n172 = Build Array(w465) -> (w464:refnum<vi>[])
        n173 = Build Array(w462) -> (w461:refnum<vi>[])
        n174 = call "Set Enable State on Multiple Controls.vi"("Enable?"=TRUE, "Controls"=w464) -> ()  [unwired: 10 in]
        n175 = call "Set Enable State on Multiple Controls.vi"("Enable?"=FALSE, "Controls"=w461) -> ()  [unwired: 10 in]
        n176 = call <vilib>:"Add State(s) to Queue__JKI_lib_State_Machine.vi"("State(s) in (\"\")"=w471) -> ("States Out"=w470:string)  [unwired: 14 in]
      }
    }
  }
  n177 = Close Python Session(session in=w3, error in=w4) -> (11:w1:errorcluster)
  n178 = call <vilib>:"General Error Handler.vi"("type of dialog (OK msg:1)"=w2, "error in (no error)"=w1) -> ()  [unwired: 9 in, 5 out]
